vi "Extract-t0.vi"(11 "data":dynamicdata(waveform)) -> (3 "Waveform":waveform(dbl))   [LabVIEW 2025]
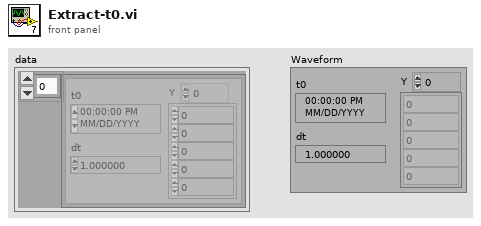
[diagram p1: front panel]
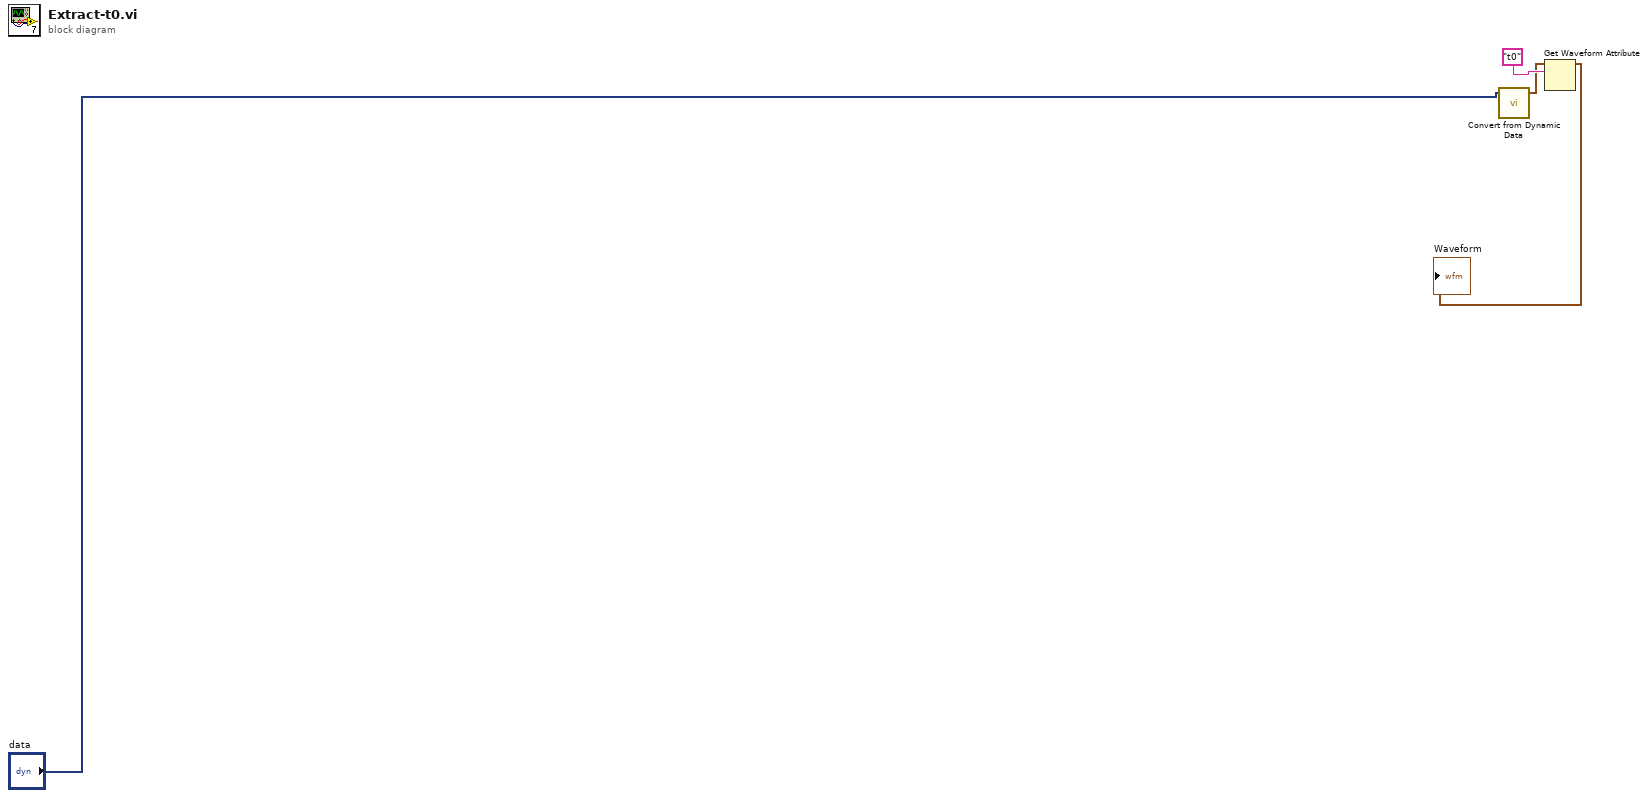
[diagram p0: block diagram]
diagram:
  n1 = call "Convert from Dynamic Data"("Dynamic Data Type"="data") -> ("Waveform"=w1:waveform(dbl))  [unwired: 3 in]
  n2 = Get Waveform Attribute(6:"t0" ("name"), 7:w1) -> (3:→"Waveform":waveform(dbl))  [unwired: 2 in, 3 out]
